vi "with_ feedback.vi"() -> ()   [LabVIEW 2017]
panel:
  out "Numeric":i32
  out "average 2":dbl
  in  "stop":bool
  out "average":dbl
  out "random num":dbl
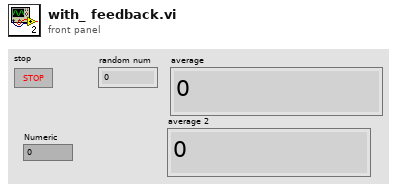
[diagram p1: front panel]
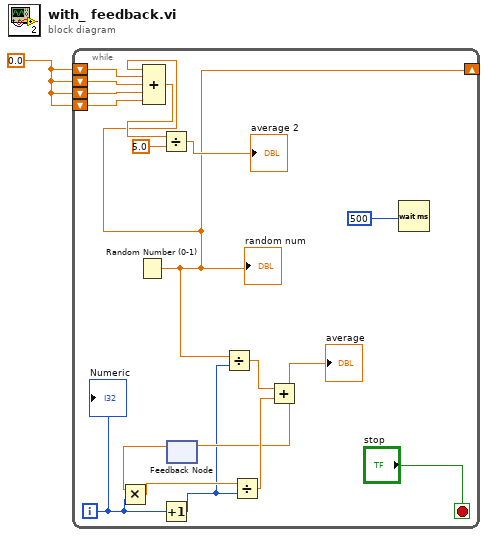
[diagram p0: block diagram]
diagram:
  w1 = 0.0 ("number: 0 to 1")
  n1 = while {
    shift-right: [w2] -> _
    shift-left: w1 -> [w9]
    shift-left: w1 -> [w8]
    shift-left: w1 -> [w7]
    shift-left: w1 -> [w6]
    i -> [w15]
    stop <- "stop" stop-if-true
    n2 = Random Number (0-1)() -> (number: 0 to 1=w2:dbl)
    "random num" <- w2
    n3 = Compound Arithmetic op=ADD(w2, w9, w8, w7, w6) -> (w5:dbl)
    n4 = Divide(x=w5, y=5.0) -> (x/y=→"average 2":dbl)
    n5 = Increment(x=w15) -> (x+1=w10:i32)
    n6 = feedback #1() -> (w16:dbl)  [unwired: 1 in]
    n7 = Multiply(x=w16, y=w15) -> (x*y=w14:dbl)
    n8 = Divide(x=w2, y=w10) -> (x/y=w17:dbl)
    n9 = Divide(x=w14, y=w10) -> (x/y=w12:dbl)
    n10 = Add(x=w17, y=w12) -> (x+y=w11:dbl)
    "average" <- w11
    n11 = feedback-in #1(w11) -> ()
    n12 = Wait (ms)(milliseconds to wait=500) -> ()  [unwired: 1 out]
    "Numeric" <- w15
  }
